vi "ScanFeedback.vi"(0 "Data IN":cluster{dbl[], dbl[], dbl[], dbl[], dbl[]}[](array[cluster]), 2 "measurement type":T1(tab), 3 "Test No.":u32) -> (1 "V breakdown":dbl, 5 "V depletion":dbl, 6 "Maximum current fluctuations":dbl, 8 "Ris [MOhm]":dbl, 9 "Cis @300V [pF/cm]":dbl)   [LabVIEW 2018]
uses:
  <vilib>/Analysis/NI_AALPro.lvlib
  <vilib>/Analysis/NI_AALBase.lvlib
panel:
  out "MEAN":dbl
  out "STD":dbl
  out "Index lin fit 1":dbl
  out "Slope":dbl
  out "capSquare1":dbl[](array[numeric])
  out "volts1":dbl[](array[numeric])
  out "volts2":dbl[](array[numeric])
  out "capSquare2":dbl[](array[numeric])
  out "deriv":dbl[](array[numeric])
  out "Slope 2":dbl
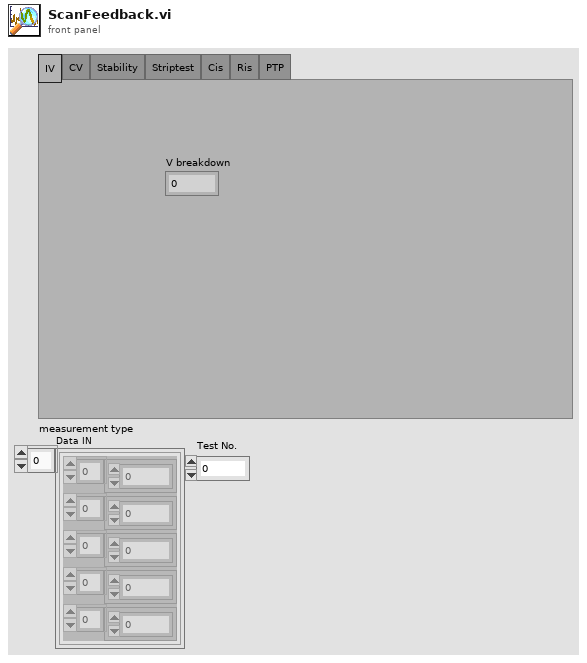
[diagram p1: front panel]
types:
  T1 = enum32{"IV", "CV", "Stability", "Striptest", "Cis", "Ris", "PTP"}
  T2 = enum16{"Reset", "Read Array", "Read Element", "Write Element", "Write Array", "Add Element", "Add Array"}
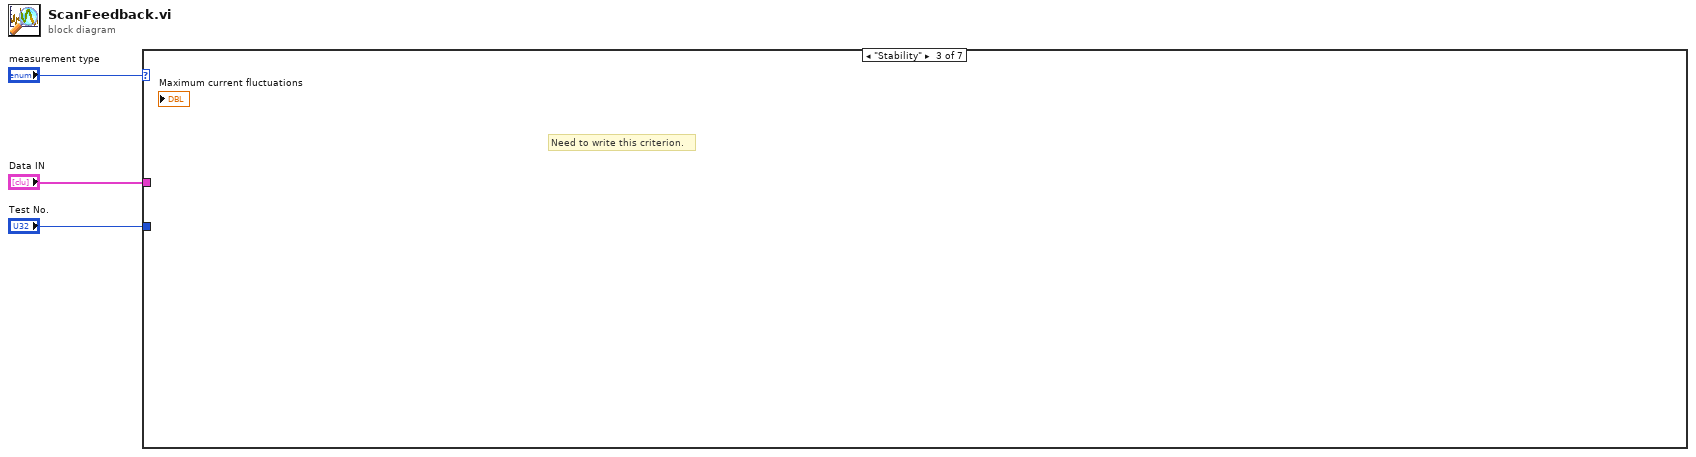
[diagram p0: block diagram]
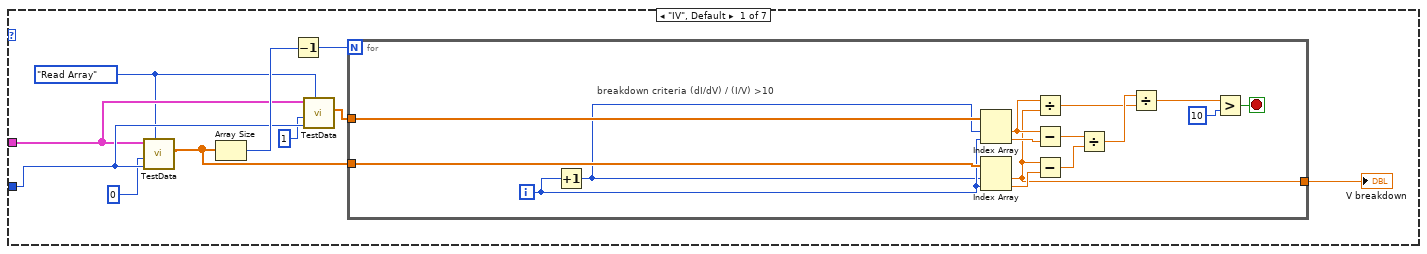
[diagram p2: hidden frame]
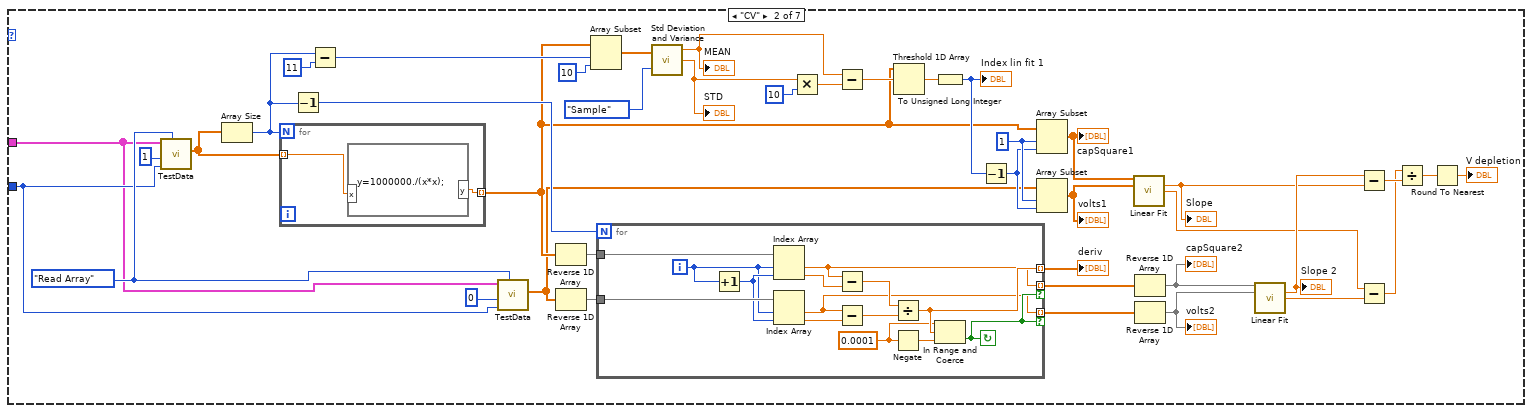
[diagram p3: hidden frame]
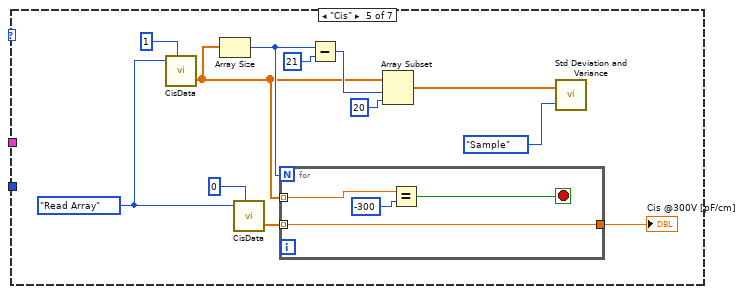
[diagram p5: hidden frame]
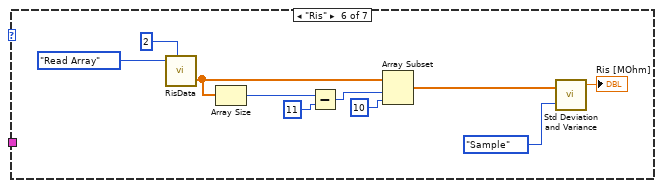
[diagram p6: hidden frame]
diagram:
  n1 = case shown="\"Stability\"" "measurement type" {
    tunnel: "Data IN" -> [w7 w31 _ _ _ _ _]
    tunnel: "Test No." -> [w10 w32 _ _ _ _ _]
    frame "IV", Default {
      w6 = enum16{"Reset", "Write Element", "Read Array"}."Read Array" ("Action")
      n2 = call "TestData.vi"("Action"=w6, "Test No."=w10, "Array No."=0, "Data IN"=w7) -> ("Array OUT"=w5:dbl[])  [unwired: 6 in, 1 out]
      n3 = Array Size(array=w5) -> (size(s)=w13:i32)
      n4 = Decrement(x=w13) -> (x-1=w12:i32)
      n5 = call "TestData.vi"("Action"=w6, "Test No."=w10, "Array No."=1, "Data IN"=w7) -> ("Array OUT"=w4:dbl[])  [unwired: 6 in, 1 out]
      n6 = for {
        N: w12 -> [_]
        tunnel: w5 -> [w27]
        tunnel: w4 -> [w28]
        tunnel: [w14] -> w11
        i -> [w24]
        stop <- w15 stop-if-true
        # "breakdown criteria (dI/dV) / (I/V) >10"
        n7 = Increment(x=w24) -> (x+1=w23:i32)
        n8 = Index Array(array=w28, index #1=w23, index #2=w24) -> (element #1=w18:dbl, element #2=w25:dbl)
        n9 = Index Array(array=w27, index #1=w23, index #2=w24) -> (element #1=w14:dbl, element #2=w26:dbl)
        n10 = Divide(x=w18, y=w14) -> (x/y=w21:dbl)
        n11 = Subtract(x=w18, y=w25) -> (x-y=w19:dbl)
        n12 = Subtract(x=w14, y=w26) -> (x-y=w20:dbl)
        n13 = Divide(x=w19, y=w20) -> (x/y=w22:dbl)
        n14 = Divide(x=w22, y=w21) -> (x/y=w16:dbl)
        n15 = Greater?(x=w16, y=10) -> (0:w15:bool)
      }
      "V breakdown" <- w11
    }
    frame "CV" {
      w35 = enum16{"Reset", "Write Element", "Read Array"}."Read Array" ("Action")
      w41 = 1
      n16 = call "TestData.vi"("Action"=w35, "Test No."=w32, "Array No."=1, "Data IN"=w31) -> ("Array OUT"=w29:dbl[])  [unwired: 6 in, 1 out]
      n17 = Array Size(array=w29) -> (size(s)=w37:i32)
      n18 = for {
        N: w37 -> [_]
        tunnel: w29 -> [w71] mode=indexing
        tunnel: [w70] -> w36 mode=indexing
        n19 = formula code="y=1000000./(x*x);"("x"=w71) -> ("y"=w70:dbl)
      }
      n20 = Decrement(x=w37) -> (x-1=w54:i32)
      n21 = Subtract(x=w37, y=11) -> (x-y=w68:i32)
      n22 = call "TestData.vi"("Action"=w35, "Test No."=w32, "Array No."=0, "Data IN"=w31) -> ("Array OUT"=w30:dbl[])  [unwired: 6 in, 1 out]
      n23 = Reverse 1D Array(array=w36) -> (reversed array=w57:dbl[])
      n24 = Reverse 1D Array(array=w30) -> (reversed array=w38:dbl[])
      n25 = Array Subset(array=w36, index=w68, length=10) -> (w66:dbl[])
      n26 = for {
        N: w54 -> [_]
        tunnel: w57 -> [w85]
        tunnel: [w78] -> w56 mode=indexing if=w79
        tunnel: [w74] -> w53 mode=indexing if=w79
        tunnel: [w82] -> w50 mode=indexing
        tunnel: w38 -> [w77]
        i -> [w75]
        stop <- w79 continue-if-true
        w80 = 0.0001
        n27 = Increment(x=w75) -> (x+1=w76:i32)
        n28 = Index Array(array=w85, index #1=w75, index #2=w76) -> (element #1=w78:dbl, element #2=w83:dbl)
        n29 = Index Array(array=w77, index #1=w75, index #2=w76) -> (element #1=w74:dbl, element #2=w73:dbl)
        n30 = Subtract(x=w78, y=w83) -> (x-y=w84:dbl)
        n31 = Subtract(x=w74, y=w73) -> (x-y=w72:dbl)
        n32 = Divide(x=w84, y=w72) -> (x/y=w82:dbl)
        n33 = Negate(x=w80) -> (-x=w81:dbl)
        n34 = In Range and Coerce(upper limit=w80, x=w82, lower limit=w81) -> (In Range?=w79:bool)  [unwired: 1 out]
      }
      "deriv" <- w50
      n35 = call <vilib>:"Std Deviation and Variance.vi"("X"=w66, "Weighting (Sample)"=enum16{"Sample", "Population"}."Sample") -> ("mean"=w62:dbl, "standard deviation"=w51:dbl)  [unwired: 1 out]
      "MEAN" <- w62
      "STD" <- w51
      n36 = Multiply(x=w51, y=10) -> (x*y=w63:dbl)
      n37 = Subtract(x=w62, y=w63) -> (x-y=w61:dbl)
      n38 = Threshold 1D Array(2:w61, 3:w36) -> (0:w60:dbl)  [unwired: 1 in]
      n39 = To Unsigned Long Integer(number=w60) -> (unsigned 32bit integer=w59:u32)
      "Index lin fit 1" <- w59
      n40 = Decrement(x=w59) -> (x-1=w40:u32)
      n41 = Array Subset(array=w36, index=w41, length=w40) -> (w58:dbl[])
      "capSquare1" <- w58
      n42 = Array Subset(array=w30, index=w41, length=w40) -> (w39:dbl[])
      "volts1" <- w39
      n43 = call <vilib>:"Linear Fit.vi"("Y"=w58, "X"=w39) -> ("slope"=w48:dbl, "intercept"=w46:dbl)  [unwired: 9 in, 3 out]
      "Slope" <- w48
      n44 = Reverse 1D Array(array=w56) -> (reversed array=w55:dbl[])
      "capSquare2" <- w55
      n45 = Reverse 1D Array(array=w53) -> (reversed array=w52:dbl[])
      "volts2" <- w52
      n46 = call <vilib>:"Linear Fit.vi"("Y"=w55, "X"=w52) -> ("slope"=w49:dbl, "intercept"=w47:dbl)  [unwired: 9 in, 3 out]
      "Slope 2" <- w49
      n47 = Subtract(x=w49, y=w48) -> (x-y=w45:dbl)
      n48 = Subtract(x=w46, y=w47) -> (x-y=w44:dbl)
      n49 = Divide(x=w44, y=w45) -> (x/y=w43:dbl)
      n50 = Round To Nearest(number=w43) -> (nearest integer value=→"V depletion":dbl)
    }
    frame "Stability" {
      # "Need to write this criterion."
    }
    frame "Striptest" {
    }
    frame "Cis" {
      w91 = T2."Read Array" ("Action")
      n51 = call "CisData.vi"("Action"=w91, "Array No."=1) -> ("Array OUT"=w88:dbl[])  [unwired: 3 in, 1 out]
      n52 = Array Size(array=w88) -> (size(s)=w89:i32)
      n53 = call "CisData.vi"("Action"=w91, "Array No."=0) -> ("Array OUT"=w87:dbl[])  [unwired: 3 in, 1 out]
      n54 = for {
        N: w89 -> [_]
        tunnel: w88 -> [w100] mode=indexing
        tunnel: w87 -> [w98] mode=indexing
        tunnel: [w98] -> w86
        stop <- w99 stop-if-true
        n55 = Equal?(x=w100, y=-300) -> (x = y?=w99:bool)
      }
      "Cis @300V [pF/cm]" <- w86
      n56 = Subtract(x=w89, y=21) -> (x-y=w93:i32)
      n57 = Array Subset(array=w88, index=w93, length=20) -> (w92:dbl[])
      n58 = call <vilib>:"Std Deviation and Variance.vi"("X"=w92, "Weighting (Sample)"=enum16{"Sample", "Population"}."Sample") -> ()  [unwired: 3 out]
    }
    frame "Ris" {
      n59 = call "RisData.vi"("Action"=T2."Read Array", "Array No."=2) -> ("Array OUT"=w102:dbl[])  [unwired: 3 in, 1 out]
      n60 = Array Size(array=w102) -> (size(s)=w110:i32)
      n61 = Subtract(x=w110, y=11) -> (x-y=w107:i32)
      n62 = Array Subset(array=w102, index=w107, length=10) -> (w106:dbl[])
      n63 = call <vilib>:"Std Deviation and Variance.vi"("X"=w106, "Weighting (Sample)"=enum16{"Sample", "Population"}."Sample") -> ("mean"=→"Ris [MOhm]":dbl)  [unwired: 2 out]
    }
    frame "PTP" {
    }
  }
